vi "_Check Offset.vi"(1 "Board":T1 items=["Quad DC Board", "Lens 1 (Slot 8) Module", "Lens 2 (Slot 6) Module", "Detector Board", "Quad DC Board with Test Points", "Lens 1 Module with Test Points", "Len 2 Module with Test Points", "", "", "", "", ""], 2 "Row#":i32, 3 "Offset In":dbl) -> (0 "Offset Out":dbl)   [LabVIEW 2012]
uses:
  Type/_Board ID.ctl
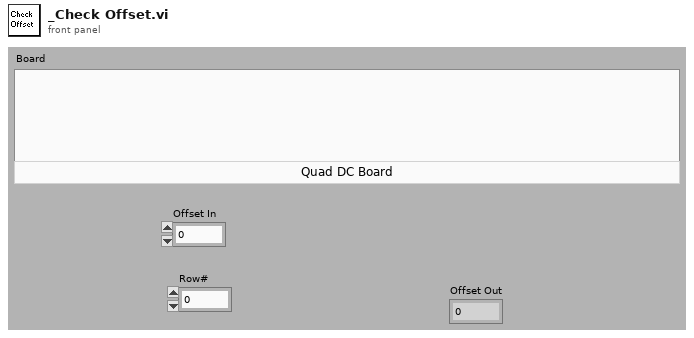
[diagram p1: front panel]
types:
  T1 = typedef "_Board ID.ctl" = u16
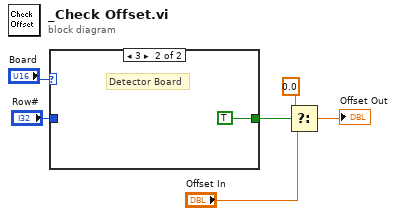
[diagram p0: block diagram]
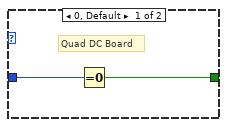
[diagram p2: hidden frame]
diagram:
  n1 = case shown="3" "Board" {
    tunnel: "Row#" -> [w8 _]
    tunnel: [w7 TRUE] -> w3
    frame 0, Default {
      # "Quad DC Board"
      n2 = Equal To 0?(x=w8) -> (x = 0?=w7:bool)
    }
    frame 3 {
      # "Detector Board"
    }
  }
  n3 = Select(t=0.0, s=w3, f="Offset In") -> (s? t:f=→"Offset Out":dbl)
